vi "Read sensor 2.vi"(8 "error in (no error)":errorcluster, 10 "Sensor value in":dbl, 11 "VISA resource name in":refnum<visa-resource-name>) -> (0 "error out":errorcluster, 2 "Sensor value out":dbl, 3 "VISA resource name out":refnum<visa-resource-name>)   [LabVIEW 2020, in "Control de MaP.lvlib"]
uses:
  Control de MaP.lvlib
  Write--command.vi
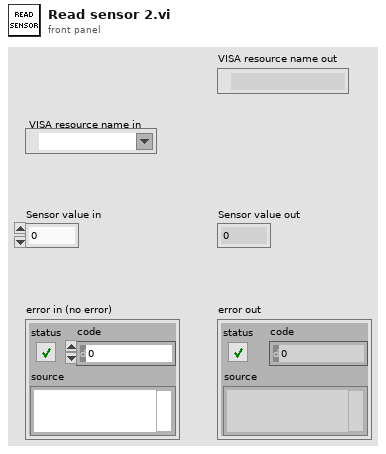
[diagram p1: front panel]
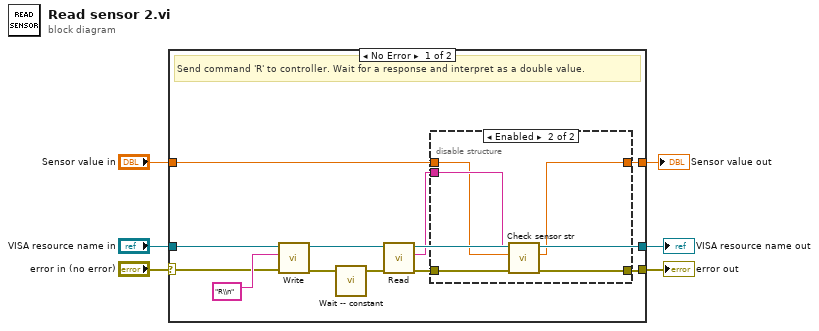
[diagram p0: block diagram]
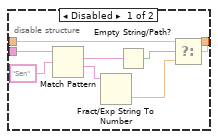
[diagram p2: hidden frame]
diagram:
  n1 = case shown="No Error" "error in (no error)" {
    selector: "error in (no error)" -> [w12 w33]
    tunnel: [w18 w34] -> w6
    tunnel: "Sensor value in" -> [w17 w34]
    tunnel: [w7 w33] -> w3
    tunnel: "VISA resource name in" -> [w11 w32]
    tunnel: [w10 w32] -> w1
    frame No Error {
      # "Send command 'R' to controller. Wait for a response and interpret as a double value."
      n2 = call-poly "Write.vi"("error in (no error)"=w12, "Command"="R\\n", "VISA resource name"=w11) -> ("error out"=w14:errorcluster, "VISA resource name out"=w15:refnum<visa-resource-name>)  [unwired: 6 in, 1 out]
      n3 = call "Wait -- constant.vi"("error in (no error)"=w14) -> ("error out"=w13:errorcluster)  [unwired: 4 in]
      n4 = call "Read.vi"("error in (no error)"=w13, "VISA resource name"=w15) -> ("error out"=w8:errorcluster, "Recibo de Datos"=w9:string, "VISA resource name out"=w10:refnum<visa-resource-name>)  [unwired: 6 in, 1 out]
      n5 = disable-structure shown="Enabled" {
        disable-tunnel: [w26 w27] -> w18
        disable-tunnel: w17 -> [w23 w28]
        disable-tunnel: w9 -> [w19 w29]
        disable-tunnel: w8 -> [_ w31]
        disable-tunnel: [_ w30] -> w7
        frame Disabled {
          n6 = Match Pattern(string=w19, regular expression="Sen") -> (match substring=w21:string, after substring=w24:string)  [unwired: 1 in, 2 out]
          n7 = Fract/Exp String To Number(string=w24) -> (number=w25:dbl)  [unwired: 3 in, 1 out]
          n8 = Empty String/Path?(string/path=w21) -> (empty?=w22:bool)
          n9 = Select(t=w23, s=w22, f=w25) -> (s? t:f=w26:dbl)
        }
        frame Enabled {
          n10 = call "Check sensor str.vi"("error in (no error)"=w31, "Sensor value in"=w28, "string"=w29) -> ("error out"=w30:errorcluster, "Sensor value out"=w27:dbl)  [unwired: 6 in]
        }
      }
    }
    frame Error {
    }
  }
  "Sensor value out" <- w6
  "error out" <- w3
  "VISA resource name out" <- w1
